vi "Main.vi"() -> ()   [LabVIEW 2019, in "DOWNLINK.lvlib"]
doc: "This template is based off of the Queued Message Handler design pattern and the Queued Message Handler project template that ships with LabVIEW.\n\nThe main difference is that the queue is private to this module and communication between modules is performed via Broadcast and Request events.\n\nRequest events are wrapped in public API methods and are handled in the Event Handling Loop (EHL) of this VI. Any module can register for Broadcast events sent by this module. The EHL generates messages based on user interface actions.\n\nThe Message Handling Loop (MHL) processes messages generated by the EHL, or by other messages. The messages are string values, so new messages can be added easily to the Message Cases case structure in the MHL. Each message cluster can also provide an optional value for Message Data, which is a variant that can be converted to whatever message-specific data is required.\n_____\nBased on Delacor QMH Project Template 4.2.1.64."
uses:
  DOWNLINK.lvlib
  <vilib>/Delacor/Delacor QMH/Libraries/Module Admin_class/Delacor_lib_QMH_Module Admin.lvclass
  UI/Visual/Visual.xctl
  TypeDef/ISO.ctl
  Module Data--cluster.ctl
  Do Something Argument--cluster.ctl
  <vilib>/Delacor/Delacor QMH/Libraries/Message Queue_class/Delacor_lib_QMH_Message Queue.lvclass/Delacor_lib_QMH_Message Queue.ctl
  Do Something Else Argument--cluster.ctl
  Do Something Else and Wait for Reply Argument--cluster.ctl
  Do Something Else and Wait (Reply Payload)--cluster.ctl
  Stop Argument--cluster.ctl
  <vilib>/Delacor/Delacor QMH/Libraries/Module Admin_class/Delacor_lib_QMH_Module Admin.lvclass/Delacor_lib_QMH_Module Admin.ctl
  CH_LINK Argument--cluster.ctl
  TypeDef/Sett data.ctl
  TypeDef/Noise.ctl
  TypeDef/Link.ctl
  Show Power Argument--cluster.ctl
  Analys Argument--cluster.ctl
  TypeDef/Analys data.ctl
  TypeDef/Analys type.ctl
  <vilib>/Utility/miscctls.llb/LVPointTypeDef.ctl
  Class/ISO 14443 A DOWN.lvclass
  Class/ISO 14443 B DOWN.lvclass
  Class/Felica DOWN.lvclass
  Class/ISO 15693 DOWN.lvclass
  <vilib>/Delacor/Delacor QMH/Libraries/Message Queue_class/Delacor_lib_QMH_Enqueue Message (Single).vi
  <vilib>/Delacor/Delacor QMH/Libraries/Module Admin_class/Delacor_lib_QMH_Get External Launch.vi
  <vilib>/Utility/error.llb/Error Cluster From Error Code.vi
  <vilib>/ErrorRing/Error Ring.xnode
  <vilib>/Delacor/Delacor QMH/Libraries/Message Queue_class/Delacor_lib_QMH_Message Queue.lvclass
  Server/Server.lvlib
panel:
  out "ISO/IEC":T1
  out "Noise attenuator":dbl(knob) scale=0.0..10.0
  out "Q":dbl(slide) scale=0.0..10.0
  out "Visual":cluster{"Notes":string[], "Frame":u8[]}(xcontrol)
  in  "Subpanel Ref":refnum<vi>
  in  "Simulate MHL Error":bool
  in  "Simulate EHL Error":bool
  out "error out":errorcluster
  in  "Module Admin":refnum<class "Delacor_lib_QMH_Module Admin.lvclass">
  out "X":dbl
  out "Status":string
  in  "Do Something Else <Replace Me>":bool
  in  "Do Something":bool
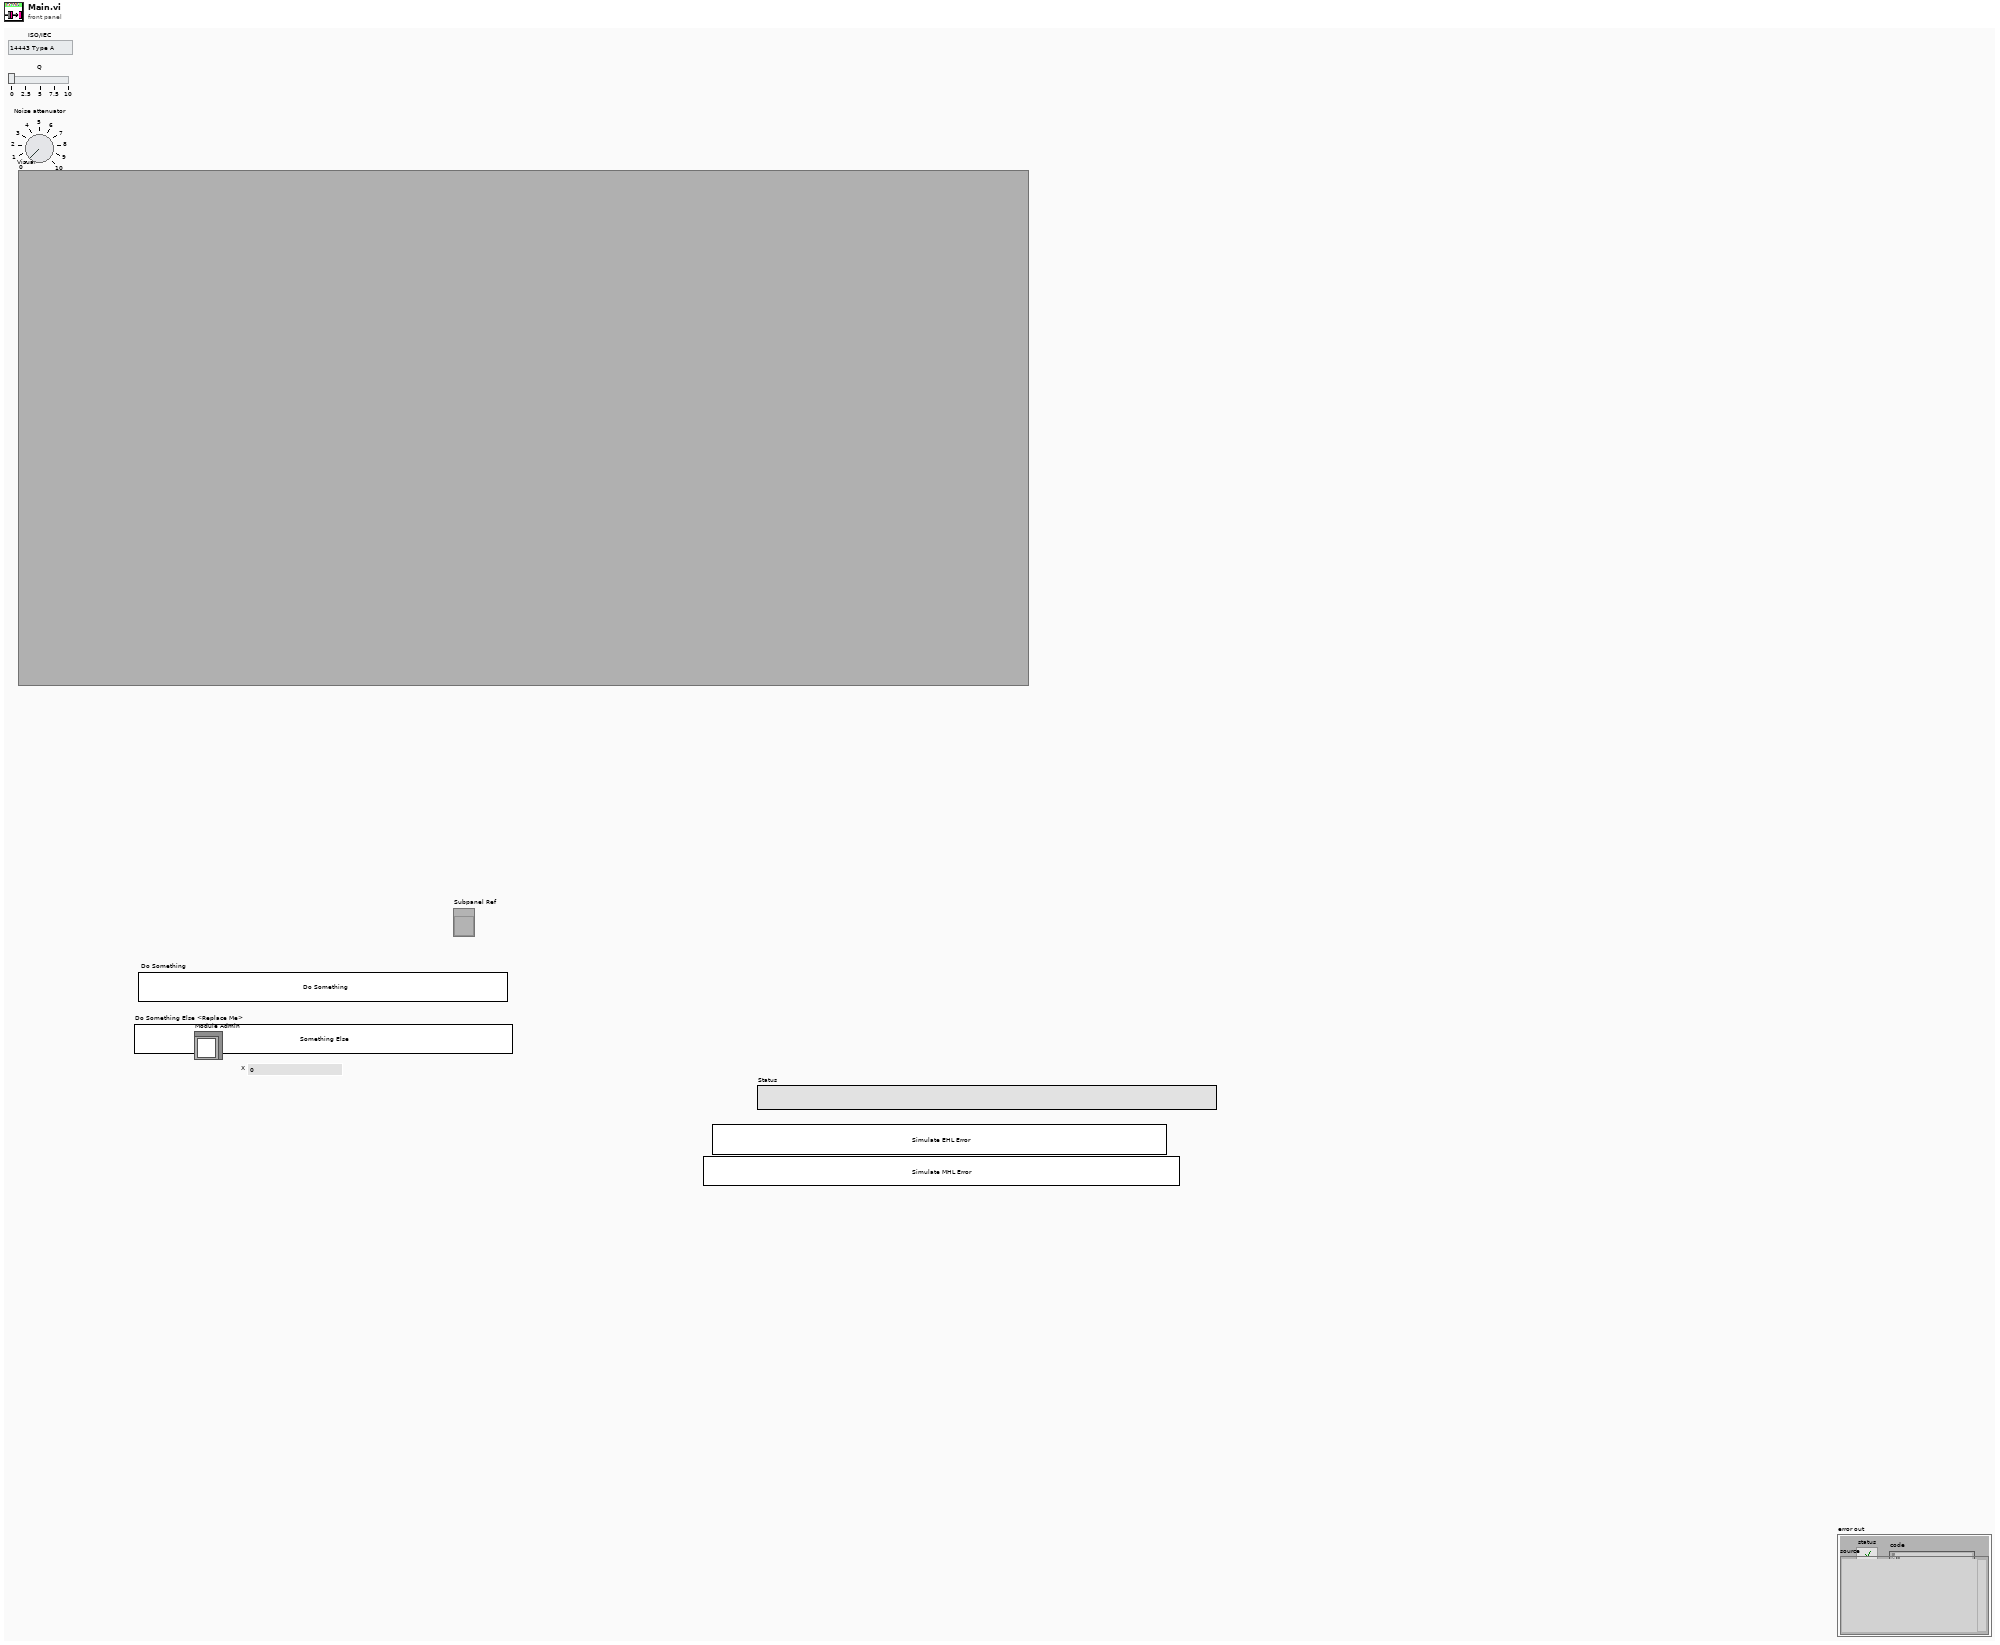
[diagram p1: front panel]
types:
  T1 = typedef "ISO.ctl" = enum16{"14443 Type A", "14443 Type B", "Felica", "15693"}
  T2 = typedef "DOWNLINK.lvlib/Request Events--cluster.ctl" = cluster{"Stop Module":refnum<user-event>, "Do Something":refnum<user-event>, "Do Something Else":refnum<user-event>, "Do Something Else and Wait for Reply":refnum<user-event>, "Show Panel":refnum<user-event>, "Hide Panel":refnum<user-event>, "Get Module Execution Status":refnum<user-event>, "Show Diagram":refnum<user-event>, "CH_LINK":refnum<user-event>, "Show Power":refnum<user-event>, "Analys":refnum<user-event>}
  T3 = typedef "Server.lvlib/Broadcast Events--cluster.ctl" = cluster{"Module Did Init":refnum<user-event>, "Status Updated":refnum<user-event>, "Error Reported":refnum<user-event>, "Did Something":refnum<user-event>, "Module Did Stop":refnum<user-event>, "Update Module Execution Status":refnum<user-event>, "Apply settings":refnum<user-event>}
  T4 = typedef "DOWNLINK.lvlib/Module Data--cluster.ctl" = cluster{"Status":string, "Power":waveform(dbl)}
  T5 = typedef "DOWNLINK.lvlib/Do Something Argument--cluster.ctl" = cluster{"Do Something Msg":string}
  T6 = typedef "DOWNLINK.lvlib/Do Something Else Argument--cluster.ctl" = cluster{"Do Something Else Msg":string, "X":dbl}
  T7 = typedef "DOWNLINK.lvlib/Do Something Else and Wait for Reply Argument--cluster.ctl" = cluster{"Do Something Else Msg":string, "X":dbl, "Wait Notifier":refnum<notifier>, "wait for reply":bool}
  T8 = enum32{"invalid lock state", "Not Locked", "Locked (No Password)", "Password-protected"}
  T9 = typedef "DOWNLINK.lvlib/Stop Argument--cluster.ctl" = cluster{"Origin":string, "Exit via Stop Module Req?":bool, "Wait for Module to stop?":bool}
  T10 = typedef "DOWNLINK.lvlib/CH_LINK Argument--cluster.ctl" = cluster{"Subpanel Ref":refnum<vi>}
  T11 = typedef "Link.ctl" = enum16{"UPLINK", "DOWNLINK"}
  T12 = typedef "Sett data.ctl" = cluster{"Filter":i32, "Gain":dbl, "Bit rate":dbl, "ISO/IEC w ":T1, "BI":cluster{"R":dbl, "C":dbl, "L":dbl}, "BM":cluster{"R":dbl, "C":dbl, "L":dbl}, "M":cluster{"Метка":i64, "Считыветель":i64}, "Type noise":T13, "Link":T11, "Noise attenuator":dbl, "Signal gain":dbl, "Distance":dbl}
  T13 = typedef "Noise.ctl" = enum16{"Гауссовский шум", "Белый шум"}
  T14 = typedef "DOWNLINK.lvlib/Show Power Argument--cluster.ctl" = cluster{"Boolean":bool}
  T15 = typedef "DOWNLINK.lvlib/Analys Argument--cluster.ctl" = cluster{"Data link":variant, "data":T16}
  T16 = typedef "Analys data.ctl" = cluster{"min attenuator":dbl, "max distanse":dbl, "num sample":dbl, "type":T17}
  T17 = typedef "Analys type.ctl" = enum16{"Noise", "Distance"}
  T18 = typedef "LVPointTypeDef.ctl" = cluster{"Horizontal":i16, "Vertical":i16}
  T19 = typedef "DOWNLINK.lvlib/Do Something Else and Wait (Reply Payload)--cluster.ctl" = cluster{"Value":dbl, "error":errorcluster}
  T20 = typedef "Visual.xctl/data.ctl" = cluster{"Notes":string[], "Frame":u8[]}
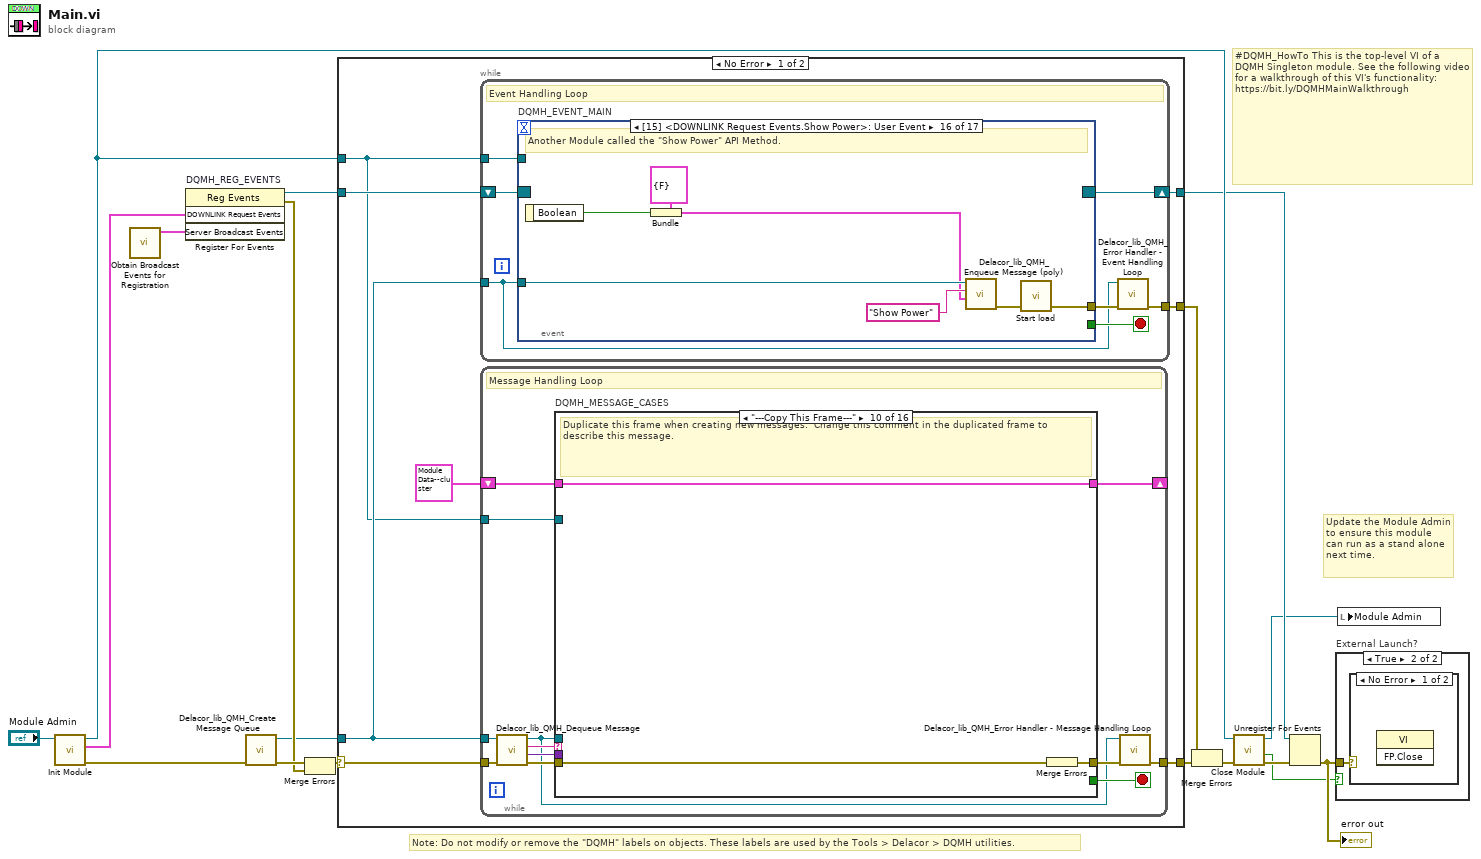
[diagram p0: block diagram]
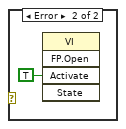
[diagram p3: hidden frame]
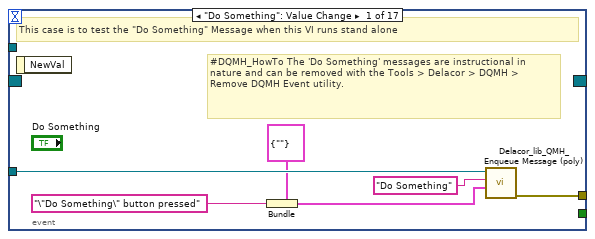
[diagram p4: hidden frame]
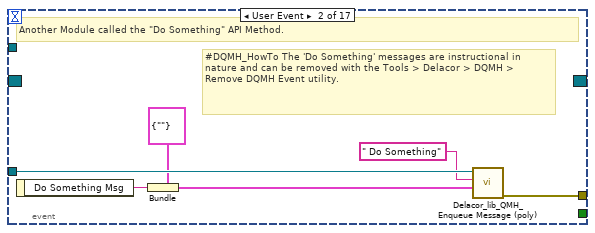
[diagram p5: hidden frame]
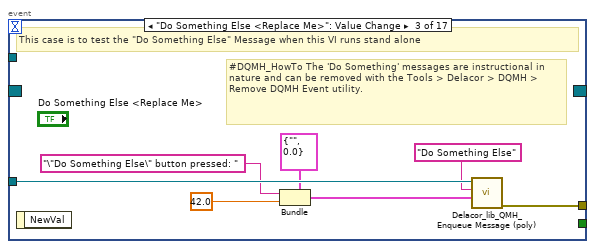
[diagram p6: hidden frame]
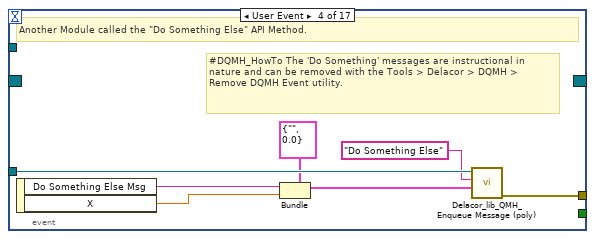
[diagram p7: hidden frame]
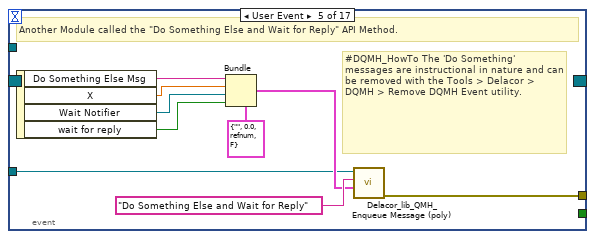
[diagram p8: hidden frame]
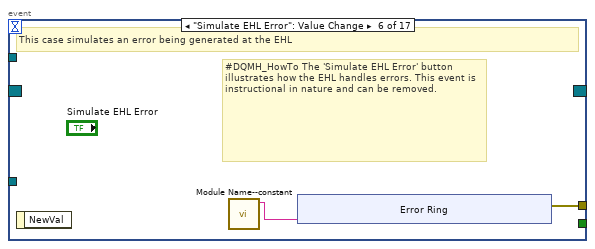
[diagram p9: hidden frame]
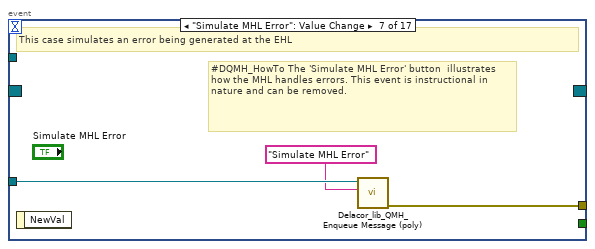
[diagram p10: hidden frame]
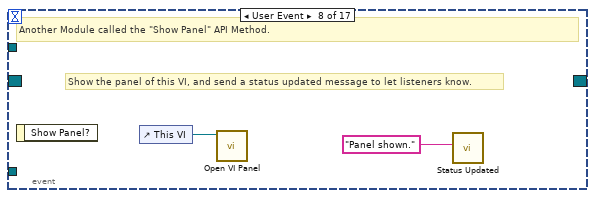
[diagram p11: hidden frame]
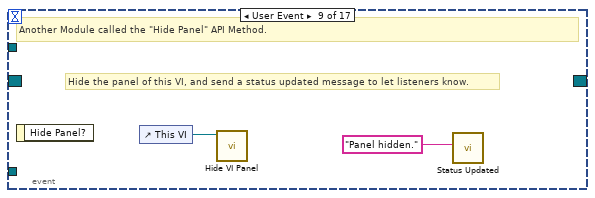
[diagram p12: hidden frame]
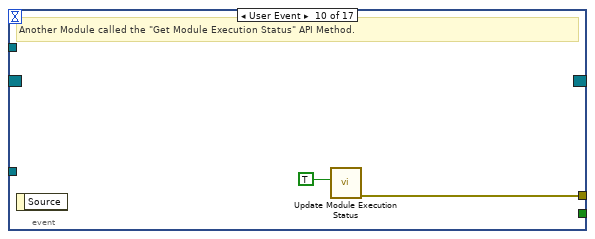
[diagram p13: hidden frame]
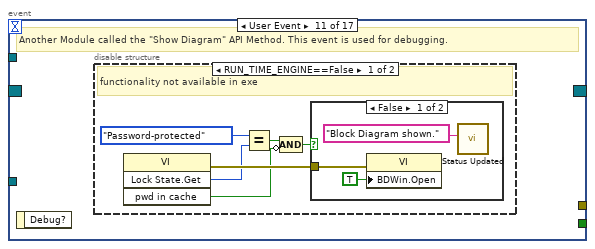
[diagram p14: hidden frame]
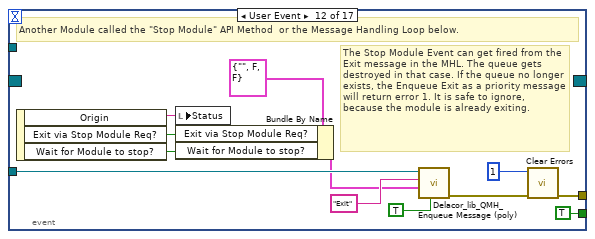
[diagram p17: hidden frame]
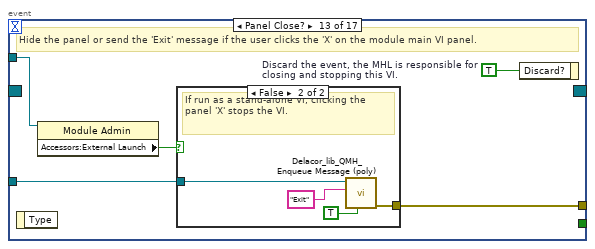
[diagram p18: hidden frame]
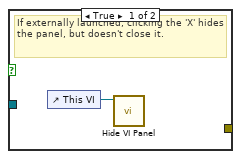
[diagram p19: hidden frame]
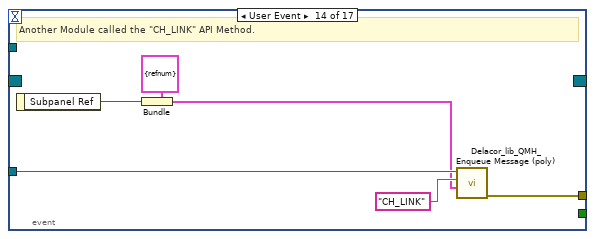
[diagram p20: hidden frame]
diagram:
  # "#DQMH_HowTo This is the top-level VI of a DQMH Singleton module. See the following video for a walkthrough of this VI's functionality: https://bit.ly/DQMHMainWalkthrough"
  # "Note: Do not modify or remove the \"DQMH\" labels on objects. These labels are used by the Tools > Delacor > DQMH utilities."
  # "Update the Module Admin to ensure this module can run as a stand alone next time."
  n1 = call "Init Module.vi"("Singleton Module Admin in"="Module Admin") -> ("error out"=w17:errorcluster, "DOWNLINK Request Events"=w6:T2, "Singleton Module Admin out"=w9:refnum<class "Delacor_lib_QMH_Module Admin.lvclass">)  [unwired: 8 in]
  n2 = call "Obtain Broadcast Events for Registration.vi"() -> ("Server Broadcast Events"=w1:T3)  [unwired: 9 in, 2 out]
  n3 = register-events "DQMH_REG_EVENTS"(w6, w1) -> (reference out=w7:refnum<event-registration>, error out=w10:errorcluster)  [unwired: 2 in]
  n4 = call <vilib>:"Delacor_lib_QMH_Create Message Queue.vi"("error in (no error)"=w17) -> ("error out"=w12:errorcluster, "Message Queue"=w5:refnum<class "Delacor_lib_QMH_Message Queue.lvclass">)  [unwired: 9 in]
  n5 = Merge Errors(w12, w10) -> (w11:errorcluster)
  n6 = case shown="No Error" w11 {
    selector: w11 -> [w24 w364]
    tunnel: [w26 w364] -> w18
    tunnel: [w23 w361] -> w8
    tunnel: w7 -> [w21 w361]
    tunnel: w5 -> [w20 _]
    tunnel: [w25 _] -> w15
    tunnel: w9 -> [w19 w357]
    frame No Error {
      n7 = while {
        tunnel: w20 -> [w27]
        shift-right: [w30] -> w23
        shift-left: w21 -> [w31]
        tunnel: [w32] -> w25
        tunnel: w19 -> [w28]
        stop <- w29 stop-if-true
        # "Event Handling Loop"
        n8 = event "DQMH_EVENT_MAIN" shown="[15] <DOWNLINK Request Events.Show Power>: User Event" {
          selector: w31 -> [_ _ _ _ _ _ _ _ _ _ _ _ _ _ _ _ _]
          dyn-events: [_ _ _ _ _ _ _ _ _ _ _ _ _ _ _ _ _] -> w30
          timeout: _ -> [_ _ _ _ _ _ _ _ _ _ _ _ _ _ _ _ _]
          tunnel: [_ _ _ _ _ _ _ _ _ _ _ TRUE ("Discard?") _ _ _ _ _] -> w29
          tunnel: w27 -> [w38 w44 w51 w58 w61 _ w79 _ _ _ _ w103 w110 w123 w126 w145 w152]
          tunnel: [w39 w45 w52 w59 w68 w70 w80 _ _ w86 _ w106 w112 w118 w124 w139 w148] -> w33
          tunnel: w28 -> [_ _ _ _ _ _ _ _ _ _ _ _ w109 _ _ _ _]
          event "Do Something": Value Change {
            # "#DQMH_HowTo The 'Do Something' messages are instructional in nature and can be removed with the Tools > Delacor > DQMH > Remove DQMH Event utility."
            # "This case is to test the \"Do Something\" Message when this VI runs stand alone"
            n9 = event-data() -> ()  [unwired: 1 in, 1 out]
            n10 = Bundle(cluster=T5 {"Do Something Msg"=""} ("Do Something Argument"), "Do Something Msg"="\"Do Something\" button pressed" ("\"Do Something\" button pressed")) -> (w34:T5)
            n11 = call-poly <vilib>:"Delacor_lib_QMH_Enqueue Message (poly).vi"("Message Data"=w34, "Message"="Do Something", "Message Queue in"=w38) -> ("error out"=w39:errorcluster)  [unwired: 7 in, 1 out]
          }
          event User Event {
            # "#DQMH_HowTo The 'Do Something' messages are instructional in nature and can be removed with the Tools > Delacor > DQMH > Remove DQMH Event utility."
            # "Another Module called the \"Do Something\" API Method."
            n12 = event-data() -> ("Do Something Msg"=w41:string)  [unwired: 1 in]
            n13 = Bundle(cluster=T5 {"Do Something Msg"=""} ("Do Something Argument"), "Do Something Msg"=w41) -> (w40:T5)
            n14 = call-poly <vilib>:"Delacor_lib_QMH_Enqueue Message (poly).vi"("Message Data"=w40, "Message"=" Do Something", "Message Queue in"=w44) -> ("error out"=w45:errorcluster)  [unwired: 7 in, 1 out]
          }
          event "Do Something Else <Replace Me>": Value Change {
            # "#DQMH_HowTo The 'Do Something' messages are instructional in nature and can be removed with the Tools > Delacor > DQMH > Remove DQMH Event utility."
            # "This case is to test the \"Do Something Else\" Message when this VI runs stand alone"
            n15 = event-data() -> ()  [unwired: 1 in, 1 out]
            n16 = Bundle(cluster=T6 {"Do Something Else Msg"="", "X"=0.0} ("Do Something Else Argument"), "Do Something Else Msg"="\"Do Something Else\" button pressed: " ("\"Do Something Else\" button pressed"), "X"=42.0) -> (w48:T6)
            n17 = call-poly <vilib>:"Delacor_lib_QMH_Enqueue Message (poly).vi"("Message Data"=w48, "Message"="Do Something Else", "Message Queue in"=w51) -> ("error out"=w52:errorcluster)  [unwired: 7 in, 1 out]
          }
          event User Event {
            # "#DQMH_HowTo The 'Do Something' messages are instructional in nature and can be removed with the Tools > Delacor > DQMH > Remove DQMH Event utility."
            # "Another Module called the \"Do Something Else\" API Method."
            n18 = event-data() -> ("Do Something Else Msg"=w54:string, "X"=w53:dbl)  [unwired: 1 in]
            n19 = Bundle(cluster=T6 {"Do Something Else Msg"="", "X"=0.0} ("Do Something Else Argument"), "Do Something Else Msg"=w54, "X"=w53) -> (w55:T6)
            n20 = call-poly <vilib>:"Delacor_lib_QMH_Enqueue Message (poly).vi"("Message Data"=w55, "Message"="Do Something Else", "Message Queue in"=w58) -> ("error out"=w59:errorcluster)  [unwired: 7 in, 1 out]
          }
          event User Event {
            # "#DQMH_HowTo The 'Do Something' messages are instructional in nature and can be removed with the Tools > Delacor > DQMH > Remove DQMH Event utility."
            # "Another Module called the \"Do Something Else and Wait for Reply\" API Method."
            n21 = event-data() -> ("Do Something Else Msg"=w64:string, "X"=w63:dbl, "Wait Notifier"=w62:refnum<notifier>, "wait for reply"=w60:bool)  [unwired: 1 in]
            n22 = Bundle(cluster=T7 {"Do Something Else Msg"="", "X"=0.0, "Wait Notifier"=refnum, "wait for reply"=FALSE} ("Do Something Else and Wait for Reply Argument"), "Do Something Else Msg"=w64, "X"=w63, "Wait Notifier"=w62, "wait for reply"=w60) -> (w65:T7)
            n23 = call-poly <vilib>:"Delacor_lib_QMH_Enqueue Message (poly).vi"("Message Data"=w65, "Message"="Do Something Else and Wait for Reply", "Message Queue in"=w61) -> ("error out"=w68:errorcluster)  [unwired: 7 in, 1 out]
          }
          event "Simulate EHL Error": Value Change {
            # "#DQMH_HowTo The 'Simulate EHL Error' button  illustrates how the EHL handles errors. This event is instructional in nature and can be removed."
            # "This case simulates an error being generated at the EHL"
            n24 = event-data() -> ()  [unwired: 1 in, 1 out]
            n25 = call "Module Name--constant.vi"() -> ("Module Name"=w69:string)  [unwired: 11 in]
            n26 = xnode "Error Ring"("parameter 0"=w69) -> ("error out"=w70:errorcluster)
          }
          event "Simulate MHL Error": Value Change {
            # "#DQMH_HowTo The 'Simulate MHL Error' button  illustrates how the MHL handles errors. This event is instructional in nature and can be removed."
            # "This case simulates an error being generated at the EHL"
            n27 = event-data() -> ()  [unwired: 1 in, 1 out]
            n28 = call-poly <vilib>:"Delacor_lib_QMH_Enqueue Message (poly).vi"("Message"="Simulate MHL Error", "Message Queue in"=w79) -> ("error out"=w80:errorcluster)  [unwired: 8 in, 1 out]
          }
          event User Event {
            # "Show the panel of this VI, and send a status updated message to let listeners know."
            # "Another Module called the \"Show Panel\" API Method."
            n29 = event-data() -> ()  [unwired: 1 in, 1 out]
            n30 = control-ref of="This VI"() -> (w82:refnum<vi>)
            n31 = call "Open VI Panel.vi"("VI"=w82) -> ()  [unwired: 10 in, 1 out]
            n32 = call "Status Updated.vi"("Status"="Panel shown." ("format string")) -> ()  [unwired: 10 in, 1 out]
          }
          event User Event {
            # "Hide the panel of this VI, and send a status updated message to let listeners know."
            # "Another Module called the \"Hide Panel\" API Method."
            n33 = event-data() -> ()  [unwired: 1 in, 1 out]
            n34 = control-ref of="This VI"() -> (w84:refnum<vi>)
            n35 = call "Hide VI Panel.vi"("VI"=w84) -> ()  [unwired: 10 in, 1 out]
            n36 = call "Status Updated.vi"("Status"="Panel hidden." ("format string")) -> ()  [unwired: 10 in, 1 out]
          }
          event User Event {
            # "Another Module called the \"Get Module Execution Status\" API Method."
            n37 = event-data() -> ()  [unwired: 1 in, 1 out]
            n38 = call "Update Module Execution Status.vi"("Running?"=TRUE) -> ("error out"=w86:errorcluster)  [unwired: 10 in]
          }
          event User Event {
            # "Another Module called the \"Show Diagram\" API Method. This event is used for debugging."
            n39 = event-data() -> ()  [unwired: 1 in, 1 out]
            n40 = disable-structure shown="RUN_TIME_ENGINE==False" {
              frame condition #0 (active) {
                # "functionality not available in exe"
                n41 = invoke class="VI" method="Lock State.Get"() -> (error out=w92:errorcluster, "Get Lock State"=w91:T8, "pwd in cache"=w88:bool)  [unwired: 4 in, 1 out]
                n42 = Equal?(x=T8."Password-protected", y=w91) -> (x = y?=w89:bool)
                n43 = Compound Arithmetic op=AND(w89, invert w88) -> (w87:bool)
                n44 = case shown="False" w87 {
                  tunnel: w92 -> [w95 _]
                  frame False {
                    n45 = property class="VI"(error in=w95, "BDWin.Open"=TRUE ("Block Diagram Window:Open")) -> ()  [unwired: 1 in, 2 out]
                    n46 = call "Status Updated.vi"("Status"="Block Diagram shown." ("format string")) -> ()  [unwired: 10 in, 1 out]
                  }
                  frame True {
                    # "Password-protected VI, and the password is not in the cache. Do not show the diagram."
                  }
                }
              }
              frame condition #1 {
              }
            }
          }
          event User Event {
            # "The Stop Module Event can get fired from the Exit message in the MHL. The queue gets destroyed in that case. If the queue no longer exists, the Enqueue Exit as a priority message will return error 1. It is safe to ignore, because the module is already exiting."
            # "Another Module called the \"Stop Module\" API Method  or the Message Handling Loop below."
            n47 = event-data() -> ("Origin"=w102:string, "Exit via Stop Module Req?"=w98:bool, "Wait for Module to stop?"=w97:bool)  [unwired: 1 in]
            n48 = local write "Status"(w102) -> ()
            n49 = Bundle By Name(cluster=T9 {"Origin"="", "Exit via Stop Module Req?"=FALSE, "Wait for Module to stop?"=FALSE} ("Stop Argument"), "Exit via Stop Module Req?"=w98, "Wait for Module to stop?"=w97) -> (w96:T9)
            n50 = call-poly <vilib>:"Delacor_lib_QMH_Enqueue Message (poly).vi"("Priority Message? (F)"=TRUE, "Message Data"=w96, "Message"="Exit", "Message Queue in"=w103) -> ("error out"=w107:errorcluster)  [unwired: 6 in, 1 out]
            n51 = call <vilib>:"Clear Errors.vi"("error in (no error)"=w107, "specific error code to clear (0: all)"=1) -> ("error out"=w106:errorcluster)  [unwired: 4 in, 1 out]
          }
          event Panel Close? {
            w111 = TRUE  # Discard the event, the MHL is responsible for closing and stopping this VI.
            # "Hide the panel or send the 'Exit' message if the user clicks the 'X' on the module main VI panel."
            n52 = event-data() -> ()  [unwired: 1 in, 1 out]
            n53 = property class="Module Admin"(reference=w109) -> ("Accessors:External Launch"=w108:bool)  [unwired: 1 in, 2 out]
            n54 = case shown="False" w108 {
              tunnel: w110 -> [_ w116]
              tunnel: [_ w117] -> w112
              frame True {
                # "If externally launched, clicking the 'X' hides the panel, but doesn't close it."
                n55 = control-ref of="This VI"() -> (w113:refnum<vi>)
                n56 = call "Hide VI Panel.vi"("VI"=w113) -> ()  [unwired: 10 in, 1 out]
              }
              frame False {
                # "If run as a stand-alone VI, clicking the panel 'X' stops the VI."
                n57 = call-poly <vilib>:"Delacor_lib_QMH_Enqueue Message (poly).vi"("Priority Message? (F)"=TRUE, "Message"="Exit", "Message Queue in"=w116) -> ("error out"=w117:errorcluster)  [unwired: 7 in, 1 out]
              }
            }
            n58 = event-data("Discard?"=w111) -> ()  [unwired: 1 in, 1 out]
          }
          event User Event {
            # "Another Module called the \"CH_LINK\" API Method."
            n59 = event-data() -> ("Subpanel Ref"=w119:refnum<vi>)  [unwired: 1 in]
            n60 = Bundle(cluster=T10 {"Subpanel Ref"=refnum} ("CH_LINK Argument"), "Subpanel Ref"=w119) -> (w120:T10)
            n61 = call-poly <vilib>:"Delacor_lib_QMH_Enqueue Message (poly).vi"("Message Data"=w120, "Message"="CH_LINK", "Message Queue in"=w123) -> ("error out"=w118:errorcluster)  [unwired: 7 in, 1 out]
          }
          event User Event {
            n62 = event-data() -> ("Data"=w125:variant)  [unwired: 1 in]
            n63 = Variant To Data(type=T12 {"Filter"=0, "Gain"=0.0, "Bit rate"=0.0, "ISO/IEC w "=enum."14443 Type A", "BI"={"R"=0.0, "C"=0.0, "L"=0.0}, "BM"={"R"=0.0, "C"=0.0, "L"=0.0}, "M"={"Метка"=4, "Считыветель"=4}, "Type noise"=enum."Гауссовский шум", "Link"=enum."UPLINK", "Noise attenuator"=0.0, "Signal gain"=1.0, "Distance"=0.0} ("Sett data"), Variant=w125) -> (data=w127:T12, error out=w132:errorcluster)  [unwired: 1 in]
            n64 = Unbundle By Name(w127) -> ("Link"=w130:T11)
            n65 = Equal?(x=w130, y=Link."DOWNLINK" ("Link")) -> (x = y?=w128:bool)
            n66 = case shown="True" w128 {
              tunnel: w132 -> [w133 w138]
              tunnel: [w133 w136] -> w124
              tunnel: w125 -> [_ w135]
              tunnel: w126 -> [_ w134]
              frame False {
              }
              frame True {
                n67 = call-poly <vilib>:"Delacor_lib_QMH_Enqueue Message (poly).vi"("error in (no error)"=w138, "Message Data"=w135, "Message"="DOWNLINK", "Message Queue in"=w134) -> ("error out"=w136:errorcluster)  [unwired: 6 in, 1 out]
              }
            }
          }
          event User Event {
            # "Another Module called the \"Show Power\" API Method."
            n68 = event-data() -> ("Boolean"=w141:bool)  [unwired: 1 in]
            n69 = Bundle(cluster=T14 {"Boolean"=FALSE} ("Show Power Argument"), "Boolean"=w141) -> (w142:T14)
            n70 = call-poly <vilib>:"Delacor_lib_QMH_Enqueue Message (poly).vi"("Message Data"=w142, "Message"="Show Power", "Message Queue in"=w145) -> ("error out"=w140:errorcluster)  [unwired: 7 in, 1 out]
            n71 = call "Start load.vi"("error in (no error)"=w140) -> ("error out"=w139:errorcluster)  [unwired: 10 in]
          }
          event User Event {
            # "Another Module called the \"Analys\" API Method."
            n72 = event-data() -> ("Data link"=w147:variant, "data"=w146:T16)  [unwired: 1 in]
            n73 = Bundle(cluster=T15 {"Data link"=variant, "data"={"min attenuator"=0.0, "max distanse"=0.0, "num sample"=0.0, "type"=enum."Noise"}} ("Analys Argument"), "Data link"=w147, "data"=w146) -> (w149:T15)
            n74 = call-poly <vilib>:"Delacor_lib_QMH_Enqueue Message (poly).vi"("Message Data"=w149, "Message"="Analys", "Message Queue in"=w152) -> ("error out"=w148:errorcluster)  [unwired: 7 in, 1 out]
          }
        }
        n75 = call-dynamic "Delacor_lib_QMH_Error Handler - Event Handling Loop.vi"("error in (no error)"=w33, "Message Queue in"=w27) -> ("dup error in"=w32:errorcluster)  [unwired: 8 in, 1 out]
      }
      n76 = while {
        tunnel: w20 -> [w155]
        shift-right: [w159] -> _
        shift-left: T4 {"Status"="", "Power"={"t0"=timestamp(0 s since 1904-01-01), "dt"=1.0, "Y"=[]}} ("Data Cluster") -> [w160]
        tunnel: w24 -> [w163]
        tunnel: [w161] -> w26
        tunnel: w19 -> [w153]
        stop <- w158 stop-if-true
        # "Message Handling Loop"
        n77 = call-dynamic "Delacor_lib_QMH_Dequeue Message.vi"("error in (no error)"=w163, "Message Queue in"=w155) -> ("error out"=w162:errorcluster, "Message Data"=w156:variant, "Message"=w157:string, "Message Queue out"=w154:refnum<class "Delacor_lib_QMH_Message Queue.lvclass">)  [unwired: 6 in]
        n78 = case "DQMH_MESSAGE_CASES" shown="\"---Copy This Frame---\"" w157 {
          selector: w157 -> [_ _ _ _ _ _ _ _ _ _ _ _ _ _ _ w344]
          tunnel: w154 -> [_ _ _ _ _ _ _ _ _ _ w291 _ _ w312 w336 _]
          tunnel: w162 -> [w177 w186 w194 w203 w222 w244 w262 w268 w284 w287 w289 w297 w302 w319 w342 w346]
          tunnel: [w166 w186 w192 w202 w221 w242 w245 w267 w271 w286 w290 w297 w301 w315 w339 w347] -> w164
          tunnel: w160 -> [w175 w185 w191 w201 w219 w243 w251 w270 w283 w285 w292 w296 w299 w314 w335 w345]
          tunnel: [w174 w185 w191 w201 w219 w243 w250 w270 w283 w285 w292 w296 w299 w314 w335 w345] -> w159
          tunnel: [_ _ _ _ _ _ _ _ _ _ _ _ _ _ w334 _] -> w158
          tunnel: w156 -> [_ _ w190 w198 w216 w241 w261 _ w282 _ _ _ _ w313 w333 _]
          tunnel: w153 -> [w169 _ _ _ _ _ _ _ _ _ _ _ _ w311 w328 _]
          frame "Initialize" {
            w170 = "Initial Message" ("Initial Message")
            # "Initialize - Any operation that needs to be done before the module can receive messages. Synchronize Caller Events.vi will inform Start Module.vi that the module has launched and is ready to receive messages. Module Did Init.vi will broadcast that the module initialized."
            n79 = call "Synchronize Caller Events.vi"("error in (no error)"=w177, "Singleton Module Admin in"=w169) -> ("error out"=w176:errorcluster)  [unwired: 8 in, 1 out]
            n80 = property class="Module Admin"(reference=w169) -> ("Accessors:External Launch"=w168:bool)  [unwired: 1 in, 2 out]
            n81 = property on="Pane" class="Pane"("Origin"=T18 {"Horizontal"=0, "Vertical"=0}) -> ()  [unwired: 2 in, 2 out]
            n82 = case shown="False" w168 {
              frame False {
                n83 = call "Module Name--constant.vi"() -> ("Module Name"=w180:string)  [unwired: 11 in]
                n84 = property class="VI"("Front Panel.Title"=w180) -> (reference out=w179:refnum<vi>)  [unwired: 2 in, 1 out]
                n85 = invoke class="VI" method="FP.Open"(reference=w179) -> (reference out=w178:refnum<vi>)  [unwired: 4 in, 4 out]
                n86 = invoke class="VI" method="FP.Center"(reference=w178) -> ()  [unwired: 2 in, 3 out]
              }
              frame True {
                n87 = call "Module Name--constant.vi"() -> ("Module Name"=w184:string)  [unwired: 11 in]
                n88 = property class="VI"("Front Panel.Title"=w184) -> (reference out=w182:refnum<vi>, error out=w183:errorcluster)  [unwired: 2 in]
                n89 = call "Insert SubPanel.vi"("error in (no error)"=w183, "VI Ref"=w182, "Subpanel Ref"="Subpanel Ref") -> ()  [unwired: 8 in, 1 out]
              }
            }
            n90 = call "Module Name--constant.vi"() -> ("Module Name"=w172:string)  [unwired: 11 in]
            n91 = call "Module Did Init.vi"("error in (no error)"=w176, "Initialized?"=TRUE, "Origin"=w172) -> ("error out"=w167:errorcluster)  [unwired: 8 in]
            n92 = Bundle By Name(cluster=w175, "Status"=w170) -> (w174:T4)
            n93 = call "Status Updated.vi"("error in (no error)"=w167, "Status"="Запуск канала считыватель -  метка") -> ("error out"=w166:errorcluster)  [unwired: 9 in]
            "Status" <- w170
          }
          frame "--- Module Specific ---" {
            # "Separator -- The following cases handle messages specific to this Module."
          }
          frame "Do Something" {
            # "#DQMH_HowTo The 'Do Something' messages are instructional in nature and can be removed with the Tools > Delacor > DQMH > Remove DQMH Event utility."
            # "Do Something - Replace this message with functionality for your own application. Note that this message also fires the \"Did Something\" broadcast event."
            n94 = Variant To Data(error in=w194, type=T5 {"Do Something Msg"=""} ("Do Something Argument"), Variant=w190) -> (data=w189:T5, error out=w193:errorcluster)
            n95 = Unbundle By Name(w189) -> ("Do Something Msg"=w187:string)
            n96 = call "Did Something.vi"("error in (no error)"=w193, "Did Something Msg"=w187) -> ("error out"=w192:errorcluster)  [unwired: 9 in]
            n97 = local write "Status"(w187) -> ()
            n98 = call "Status Updated.vi"("Status"=w187) -> ()  [unwired: 10 in, 1 out]
          }
          frame "Do Something Else" {
            # "#DQMH_HowTo The 'Do Something' messages are instructional in nature and can be removed with the Tools > Delacor > DQMH > Remove DQMH Event utility."
            # "Do Something Else - Replace this message with functionality for your own application."
            n99 = Variant To Data(error in=w203, type=T6 {"Do Something Else Msg"="", "X"=0.0} ("Do Something Else Argument"), Variant=w198) -> (data=w199:T6, error out=w202:errorcluster)
            n100 = Unbundle By Name(w199) -> ("Do Something Else Msg"=w197:string, "X"=w196:dbl)
            "X" <- w196
            n101 = Format Into String(initial string=w197, w196) -> (resulting string=w195:string)  [unwired: 2 in, 1 out]
            n102 = local write "Status"(w195) -> ()
            n103 = call "Status Updated.vi"("Status"=w195) -> ()  [unwired: 10 in, 1 out]
          }
          frame "Do Something Else and Wait for Reply" {
            w211 = "X(%.2f)+Offset(%.2f)=%.2f"  # status message format string
            # "#DQMH_HowTo The 'Do Something' messages are instructional in nature and can be removed."
            # "Send back X with a random offset"
            # "Do Something Else and Wait for Reply - Replace this message with functionality for your own application. Note that this message must fire a notifier to let callers know it has finished execution, and it returns an error if the 'Value' is negative."
            n104 = Random Number (0-1)() -> (number: 0 to 1=w213:dbl)
            n105 = Variant To Data(error in=w222, type=T7 {"Do Something Else Msg"="", "X"=0.0, "Wait Notifier"=refnum, "wait for reply"=FALSE} ("Do Something Else and Wait for Reply Argument"), Variant=w216) -> (data=w217:T7, error out=w220:errorcluster)
            n106 = Unbundle By Name(w217) -> ("Wait Notifier"=w204:refnum<notifier>, "Do Something Else Msg"=w215:string, "X"=w212:dbl, "wait for reply"=w208:bool)
            n107 = Add(x=w213, y=w212) -> (x+y=w207:dbl)
            n108 = local write "X"(w212) -> ()
            n109 = Less Than 0?(x=w207) -> (x < 0?=w210:bool)
            n110 = Format Into String(format string=w211, initial string=w215, w212, w213, w207) -> (resulting string=w209:string)  [unwired: 1 in, 1 out]
            n111 = case shown="True" w210 {
              tunnel: [_ w229] -> w205
              frame False {
              }
              frame True {
                n112 = xnode "Error Ring"() -> ("error out"=w229:errorcluster)
              }
            }
            n113 = Bundle By Name(cluster=T19 {"Value"=0.0, "error"={"status"=FALSE, "code"=0, "source"=""}} ("notification"), "error"=w205, "Value"=w207) -> (w206:T19)
            n114 = local write "Status"(w209) -> ()
            n115 = call "Status Updated.vi"("Status"=w209) -> ()  [unwired: 10 in, 1 out]
            n116 = case shown="True" w208 {
              tunnel: w206 -> [_ w225]
              tunnel: w204 -> [_ w224]
              frame False {
              }
              frame True {
                # "Simulate an operation that requires a wait."
                n117 = flat-sequence {
                  tunnel: w225 -> [w228]
                  tunnel: w224 -> [w227]
                  tunnel: w223 -> [_]
                  frame #0 {
                    n118 = Send Notification(notification=w228, notifier=w227) -> ()  [unwired: 1 in, 2 out]
                  }
                }
                n119 = Wait (ms)(milliseconds to wait=u32 1000) -> (millisecond timer value=w223:u32)
              }
            }
            n120 = Merge Errors(w220, w205) -> (w221:errorcluster)
          }
          frame "CH_LINK" {
            # "#CodeNeeded\n1. Configure this Message Case for handling the \"CH_LINK\" message.\n2. Delete or edit this label when done."
            # "Change link in Server VI"
            n121 = Variant To Data(error in=w244, type=T10 {"Subpanel Ref"=refnum} ("CH_LINK Argument"), Variant=w241) -> (data=w239:T10, error out=w242:errorcluster)
            n122 = Unbundle By Name(w239) -> ("Subpanel Ref"=w235:refnum<vi>)
            n123 = call "Module Name--constant.vi"() -> ("Module Name"=w238:string)  [unwired: 11 in]
            n124 = property class="VI"("Front Panel.Title"=w238) -> (reference out=w236:refnum<vi>, error out=w237:errorcluster)  [unwired: 2 in]
            n125 = call "Insert SubPanel.vi"("error in (no error)"=w237, "VI Ref"=w236, "Subpanel Ref"=w235) -> ()  [unwired: 8 in, 1 out]
          }
          frame "DOWNLINK" {
            n126 = Variant To Data(error in=w262, type=T12 {"Filter"=0, "Gain"=0.0, "Bit rate"=0.0, "ISO/IEC w "=enum."14443 Type A", "BI"={"R"=0.0, "C"=0.0, "L"=0.0}, "BM"={"R"=0.0, "C"=0.0, "L"=0.0}, "M"={"Метка"=4, "Считыветель"=4}, "Type noise"=enum."Гауссовский шум", "Link"=enum."UPLINK", "Noise attenuator"=0.0, "Signal gain"=1.0, "Distance"=0.0} ("Sett data"), Variant=w261) -> (data=w254:T12, error out=w248:errorcluster)
            n127 = Unbundle By Name(w254) -> ("ISO/IEC w"=w258:T1)
            n128 = call "Start load.vi"("error in (no error)"=w248) -> ("error out"=w247:errorcluster)  [unwired: 10 in]
            n129 = case shown="\"14443 Type B\"" w258 {
              tunnel: [refnum<class "ISO 14443 A DOWN.lvclass"> refnum ("ISO 14443 A DOWN.lvclass") refnum<class "ISO 14443 B DOWN.lvclass"> refnum ("ISO 14443 B DOWN.lvclass") refnum<class "Felica DOWN.lvclass"> refnum ("Felica DOWN.lvclass") refnum<class "ISO 15693 DOWN.lvclass"> refnum ("ISO 15693 DOWN.lvclass")] -> w260
              frame "14443 Type A", Default {
              }
              frame "14443 Type B" {
              }
              frame "Felica" {
              }
              frame "15693" {
              }
            }
            n130 = call "OOP_DOWN.vi"("error in (no error)"=w247, "Sett data"=w254, "RFID system.lvclass"=w260) -> ("error out"=w257:errorcluster, "Error on  byte"=w253:dbl, "Visual"=→"Visual":T20, "Power out"=w249:waveform(dbl))  [unwired: 5 in]
            n131 = Format Into String(format string="Произведен расчет канала.\nВероятность ошибки на бит составляет: %#.3f", w253) -> (resulting string=w256:string)  [unwired: 2 in, 1 out]
            n132 = Bundle By Name(cluster=w251, "Power"=w249) -> (w250:T4)
            n133 = call "Status Updated.vi"("error in (no error)"=w257, "Status"=w256) -> ("error out"=w246:errorcluster)  [unwired: 9 in]
            n134 = call "Stop load.vi"("error in (no error)"=w246) -> ("error out"=w245:errorcluster)  [unwired: 10 in]
          }
          frame "Show Power" {
            # "Show chart with power in alone window"
            n135 = call "Stop load.vi"("error in (no error)"=w268) -> ("error out"=w267:errorcluster)  [unwired: 10 in]
            n136 = Unbundle By Name(w270) -> ("Power"=w269:waveform(dbl))
            n137 = call "Power.vi"("power wave in"=w269) -> ()  [unwired: 2 in]
          }
          frame "Analys" {
            # "Run analys of error on bit"
            n138 = Variant To Data(error in=w284, type=T15 {"Data link"=variant, "data"={"min attenuator"=0.0, "max distanse"=0.0, "num sample"=0.0, "type"=enum."Noise"}} ("Analys Argument"), Variant=w282) -> (data=w280:T15, error out=w274:errorcluster)
            n139 = call "Start load.vi"("error in (no error)"=w274) -> ("error out"=w273:errorcluster)  [unwired: 10 in]
            n140 = call "Status Updated.vi"("error in (no error)"=w273, "Status"="Запуск анализа") -> ("error out"=w277:errorcluster)  [unwired: 9 in]
            n141 = call "Analys DOWN.vi"("error in"=w277, "data"=w280) -> ("error out"=w275:errorcluster, "output cluster"=w279:cluster{"Array":dbl[], "Array":dbl[]})  [unwired: 8 in]
            n142 = call "Analys Chart.vi"("error in (no error)"=w275, "error wave in"=w279) -> ()  [unwired: 3 in]
            n143 = call "Status Updated.vi"("error in (no error)"=w275, "Status"="Окончание анализа") -> ("error out"=w272:errorcluster)  [unwired: 9 in]
            n144 = call "Stop load.vi"("error in (no error)"=w272) -> ("error out"=w271:errorcluster)  [unwired: 10 in]
          }
          frame "---Copy This Frame---" {
            # "Duplicate this frame when creating new messages.  Change this comment in the duplicated frame to describe this message."
            n145 = Merge Errors(w287) -> (w286:errorcluster)
          }
          frame "Constant IN" {
            n146 = One Button Dialog(message="Constant IN") -> ()  [unwired: 1 in, 1 out]
            n147 = disable-structure shown="Disabled" {
              disable-tunnel: w291 -> [w295 _]
              disable-tunnel: [w294 _] -> w290
              disable-tunnel: w289 -> [w293 _]
              frame Disabled {
                n148 = call-poly <vilib>:"Delacor_lib_QMH_Enqueue Message (poly).vi"("error in (no error)"=w293, "Message Queue in"=w295) -> ("error out"=w294:errorcluster)  [unwired: 8 in, 1 out]
              }
              frame Enabled {
              }
            }
          }
          frame "--- Exit and Error Handling---" {
            # "Separator - The following cases handle errors and exit messages."
          }
          frame "Simulate MHL Error" {
            # "#DQMH_HowTo The 'Simulate MHL Error' button  illustrates how the MHL handles errors. This event is instructional in nature and can be removed."
            # "Simulate an error occurring at the MHL"
            n149 = call "Module Name--constant.vi"() -> ("Module Name"=w298:string)  [unwired: 11 in]
            n150 = xnode "Error Ring"("parameter 0"=w298) -> ("error out"=w300:errorcluster)
            n151 = Merge Errors(w302, w300) -> (w301:errorcluster)
          }
          frame "Error" {
            # "Error - Check the error message data and respond accordingly. This message is sent by the \"Error Handler\" VIs at the end of each loop in this application."
            n152 = property class="Module Admin"(reference=w311) -> ("Accessors:External Launch"=w310:bool)  [unwired: 1 in, 2 out]
            n153 = Variant To Data(error in=w319, type=errorcluster {"status"=FALSE, "code"=0, "source"=""} ("error constant"), Variant=w313) -> (data=w320:errorcluster, error out=w317:errorcluster)
            n154 = call "Error Reported.vi"("Error"=w320) -> ()  [unwired: 10 in, 1 out]
            n155 = case shown="False" w310 {
              tunnel: [w325 _] -> w316
              tunnel: w312 -> [w323 _]
              tunnel: w320 -> [w324 _]
              frame False {
                # "If the module is running standalone, then pop up an error dialog and call the \"Exit\" message."
                n156 = call <vilib>:"Simple Error Handler.vi"("error in (no error)"=w324) -> ()  [unwired: 4 in, 5 out]
                n157 = call-poly <vilib>:"Delacor_lib_QMH_Enqueue Message (poly).vi"("Priority Message? (F)"=TRUE, "Message"="Exit", "Message Queue in"=w323) -> ("error out"=w325:errorcluster)  [unwired: 7 in, 1 out]
              }
              frame True {
                n158 = call "Status Updated.vi"("Status"="Ошибка модуля DOWNLINK") -> ()  [unwired: 10 in, 1 out]
              }
            }
            n159 = Merge Errors(w317, w316) -> (w315:errorcluster)
            n160 = local write "error out"(w315) -> ()
          }
          frame "Exit" {
            w332 = 91  # 91: not all Exit messages will have an argument
            w334 = TRUE  # Stop the VI
            # "Release the message queue reference"
            # "Exit - Exit the application."
            n161 = Variant To Data(error in=w342, type=T9 {"Origin"="", "Exit via Stop Module Req?"=FALSE, "Wait for Module to stop?"=FALSE} ("Stop Argument"), Variant=w333) -> (data=w330:T9, error out=w338:errorcluster)
            n162 = call <vilib>:"Clear Errors.vi"("error in (no error)"=w338, "specific error code to clear (0: all)"=w332) -> ("error out"=w341:errorcluster)  [unwired: 4 in, 1 out]
            n163 = control-ref of="This VI"() -> (w329:refnum<vi>)
            n164 = call "Status Updated.vi"("Status"="Запуск канала считыватель - метка") -> ()  [unwired: 10 in, 1 out]
            n165 = call-dynamic "Delacor_lib_QMH_Release Message Queue.vi"("error in (no error)"=w341, "Message Queue"=w336) -> ("error out"=w340:errorcluster)  [unwired: 9 in]
            n166 = call "Handle Exit.vi"("Stop Argument"=w330, "Admin in"=w328, "VI reference"=w329) -> ("error out"=w337:errorcluster)  [unwired: 7 in, 1 out]
            n167 = Merge Errors(w340, w337) -> (w339:errorcluster)
          }
          frame Default {
            # "'Default' case only runs if there is a message that isn't defined in any of the other cases.  Output a programming error."
            n168 = call "Module Name--constant.vi"() -> ("Module Name"=w343:string)  [unwired: 11 in]
            n169 = xnode "Error Ring"("parameter 0"=w344, "parameter 1"=w343) -> ("error out"=w348:errorcluster)
            n170 = Merge Errors(w346, w348) -> (w347:errorcluster)
          }
        }
        n171 = call-dynamic "Delacor_lib_QMH_Error Handler - Message Handling Loop.vi"("error in (no error)"=w164, "Message Queue in"=w154) -> ("dup error in"=w161:errorcluster)  [unwired: 8 in, 1 out]
      }
    }
    frame Error {
      # "Synchronize Caller Events.vi will inform Start Module.vi that the module has launched and will let the code calling Start Module.vi register for broadcasts and would permit the caller receive the broadcast that an error occurred at launch time."
      n172 = call "Synchronize Caller Events.vi"("Singleton Module Admin in"=w357) -> ("error out"=w362:errorcluster)  [unwired: 9 in, 1 out]
      n173 = call "Module Name--constant.vi"() -> ("Module Name"=w360:string)  [unwired: 11 in]
      n174 = Format Into String(format string="An error occurred during initialization. %s is no longer running.", w360) -> (resulting string=w358:string)  [unwired: 2 in, 1 out]
      n175 = Merge Errors(w364, w362) -> (w363:errorcluster)
      n176 = call "Error Reported.vi"("Additional Information"=w358, "Error"=w363) -> ()  [unwired: 9 in, 1 out]
    }
  }
  n177 = Merge Errors(w15, w18) -> (w14:errorcluster)
  n178 = call "Close Module.vi"("error in (no error)"=w14, "Module Admin in"=w9) -> ("error out"=w16:errorcluster, "External Launch"=w2:bool, "Module Admin out"=w3:refnum<class "Delacor_lib_QMH_Module Admin.lvclass">)  [unwired: 7 in]
  n179 = Unregister For Events(event registration refnum=w8, error in=w16) -> (error out=w13:errorcluster)
  "error out" <- w13
  n180 = case "External Launch?" shown="True" w2 {
    tunnel: w13 -> [_ w365]
    frame False {
    }
    frame True {
      n181 = case shown="No Error" w365 {
        frame No Error {
          n182 = invoke class="VI" method="FP.Close"() -> ()  [unwired: 3 in, 3 out]
        }
        frame Error {
          n183 = invoke class="VI" method="FP.Open"("Activate"=TRUE ("Activate?")) -> ()  [unwired: 4 in, 5 out]
        }
      }
    }
  }
  n184 = local write "Module Admin"(w3) -> ()
